vi "ParseRedLionReply.vi"(2 "Parameter Iidicator":string, 3 "Status Indicator":string, 4 "Red Lion String":string) -> (0 "Type":i16, 1 "Array":dbl[](array[numeric]))   [LabVIEW 2009]
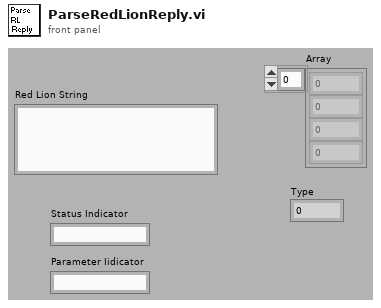
[diagram p1: front panel]
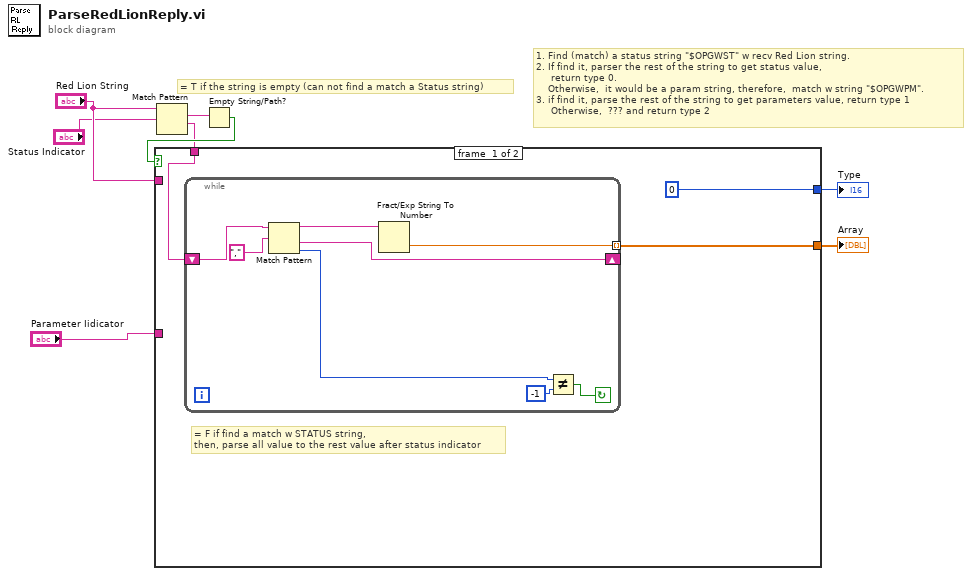
[diagram p0: block diagram]
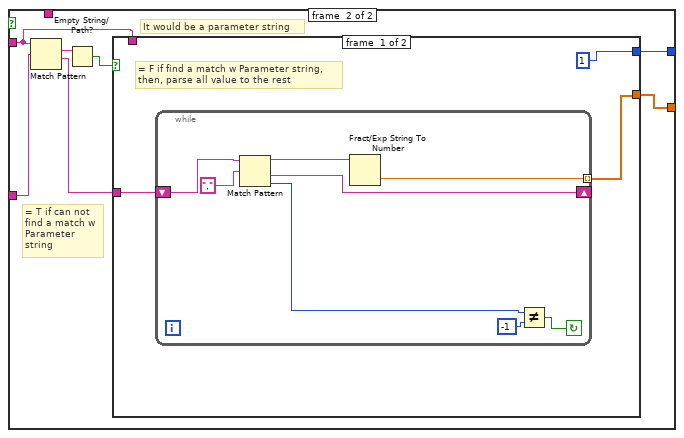
[diagram p2: hidden frame]
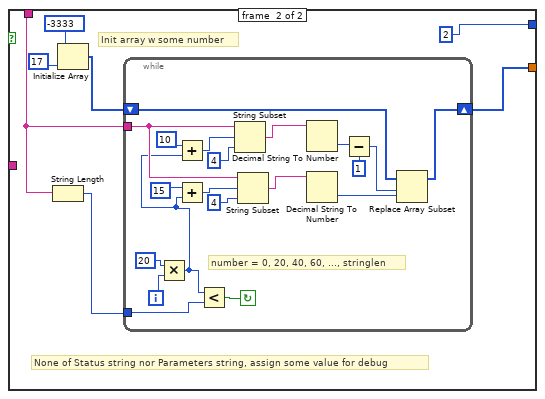
[diagram p3: hidden frame]
diagram:
  # "1. Find (match) a status string \"$OPGWST\" w recv Red Lion string.\n2. If find it, parser the rest of the string to get status value, \n     return type 0.\n    Otherwise,  it would be a param string, therefore,  match w string \"$OPGWPM\".\n3. if find it, parse the rest of the string to get parameters value, return type 1\n     Otherwise,  ??? and return type 2"
  # "= T if the string is empty (can not find a match a Status string)"
  n1 = Match Pattern(string="Red Lion String", regular expression="Status Indicator") -> (match substring=w8:string, after substring=w3:string)  [unwired: 1 in, 2 out]
  n2 = Empty String/Path?(string/path=w8) -> (empty?=w7:bool)
  n3 = case shown="True" w7 {
    tunnel: "Red Lion String" -> [_ w21]
    tunnel: "Parameter Iidicator" -> [_ w25]
    tunnel: w3 -> [w11 _]
    tunnel: [w10 w23] -> w2
    tunnel: [0 w22] -> w1
    frame #0 {
      # "= F if find a match w STATUS string,\nthen, parse all value to the rest value after status indicator"
      n4 = while {
        tunnel: [w14] -> w10 mode=indexing
        shift-right: [w13] -> _
        shift-left: w11 -> [w12]
        stop <- w16 continue-if-true
        n5 = Match Pattern(string=w12, regular expression=",") -> (before substring=w15:string, after substring=w13:string, offset past match=w17:i32)  [unwired: 1 in, 1 out]
        n6 = Fract/Exp String To Number(string=w15) -> (number=w14:dbl)  [unwired: 3 in, 1 out]
        n7 = Not Equal?(x=w17, y=-1) -> (x != y?=w16:bool)
      }
    }
    frame #1 {
      # "It would be a parameter string"
      # "= T if can not\nfind a match w\nParameter\nstring"
      n8 = Match Pattern(string=w21, regular expression=w25) -> (match substring=w26:string, after substring=w20:string)  [unwired: 1 in, 2 out]
      n9 = Empty String/Path?(string/path=w26) -> (empty?=w24:bool)
      n10 = case shown="True" w24 {
        tunnel: w21 -> [_ w40]
        tunnel: [w27 w39] -> w23
        tunnel: [1 2] -> w22
        tunnel: w20 -> [w28 _]
        frame #0 {
          # "= F if find a match w Parameter string,\nthen, parse all value to the rest"
          n11 = while {
            tunnel: [w32] -> w27 mode=indexing
            shift-right: [w31] -> _
            shift-left: w28 -> [w30]
            stop <- w34 continue-if-true
            n12 = Match Pattern(string=w30, regular expression=",") -> (before substring=w33:string, after substring=w31:string, offset past match=w35:i32)  [unwired: 1 in, 1 out]
            n13 = Fract/Exp String To Number(string=w33) -> (number=w32:dbl)  [unwired: 3 in, 1 out]
            n14 = Not Equal?(x=w35, y=-1) -> (x != y?=w34:bool)
          }
        }
        frame #1 {
          # "None of Status string nor Parameters string, assign some value for debug"
          # "Init array w some number"
          n15 = String Length(string=w40) -> (length=w43:i32)
          n16 = Initialize Array(-3333, 17) -> (w44:i32[])
          n17 = while {
            tunnel: w40 -> [w56]
            tunnel: w43 -> [w51]
            shift-right: [w49] -> w39
            shift-left: w44 -> [w48]
            i -> [w63]
            stop <- w50 continue-if-true
            # "number = 0, 20, 40, 60, ..., stringlen"
            n18 = Multiply(x=20, y=w63) -> (x*y=w52:i32)
            n19 = Add(x=10, y=w52) -> (x+y=w60:i32)
            n20 = Add(x=15, y=w52) -> (x+y=w58:i32)
            n21 = Less?(x=w52, y=w51) -> (x < y?=w50:bool)
            n22 = String Subset(string=w56, offset (0)=w60, length (rest)=4) -> (substring=w55:string)
            n23 = String Subset(string=w56, offset (0)=w58, length (rest)=4) -> (substring=w54:string)
            n24 = Decimal String To Number(string=w55) -> (number=w47:i32)  [unwired: 2 in, 1 out]
            n25 = Decimal String To Number(string=w54) -> (number=w53:i32)  [unwired: 2 in, 1 out]
            n26 = Subtract(x=w47, y=1) -> (x-y=w46:i32)
            n27 = Replace Array Subset(array=w48, new element=w53, index=w46) -> (w49:i32[])
          }
        }
      }
    }
  }
  "Array" <- w2
  "Type" <- w1
